vi "03 DPT Channel Tester.vi"() -> ()   [LabVIEW 2009]
uses:
  Hybrid Water Heater/Experiments/Sensor.ctl
  Global Test Variables DPT.vi
  <vilib>/Analysis/NI_AALBase.lvlib
panel:
  out "Output Data (Numbers Only)":dbl[](array[numeric]) format="%.2e"
  in  "Panel 4":T1[][](array[typedef])=[[{"Mean"=0.0, " St Dev."=0.0, "Color Box"=8585007}, {"Mean"=0.0, " St Dev."=0.0, "Color Box"=8585007}, {"Mean"=0.0, " St Dev."=0.0, "Color Box"=8585007}, {"Mean"=0.0, " St Dev."=0.0, "Color Box"=8585007}, {"Mean"=0.0, " St Dev."=0.0, "Color Box"=8585007}, {"Mean"=0.0, " St Dev."=0.0, "Color Box"=8585007}], [{"Mean"=0.0, " St Dev."=0.0, "Color Box"=8585007}, {"Mean"=0.0, " St Dev."=0.0, "Color Box"=8585007}, {"Mean"=0.0, " St Dev."=0.0, "Color Box"=8585007}, {"Mean"=0.0, " St Dev."=0.0, "Color Box"=8585007}, {"Mean"=0.0, " St Dev."=0.0, "Color Box"=8585007}, {"Mean"=0.0, " St Dev."=0.0, "Color Box"=8585007}], [{"Mean"=0.0, " St Dev."=0.0, "Color Box"=8585007}, {"Mean"=0.0, " St Dev."=0.0, "Color Box"=8585007}, {"Mean"=0.0, " St Dev."=0.0, "Color Box"=8585007}, {"Mean"=0.0, " St Dev."=0.0, "Color Box"=8585007}, {"Mean"=0.0, " St Dev."=0.0, "Color Box"=8585007}, {"Mean"=0.0, " St Dev."=0.0, "Color Box"=8585007}]]
  in  "Agilent Reference":refnum<visa-resource-name>="AGILENT-34980A"
  in  "Analog Min OK":dbl=100.0
  in  "Analog Max OK":dbl=400.0
  in  "StDev Thresh":dbl=0.2
  in  "TC Min OK Val":dbl=20.0
  in  "TC Max OK Val":dbl=400.0
  out "Analog":T1[](array[typedef])=[{"Mean"=0.0, " St Dev."=0.0, "Color Box"=8585007}, {"Mean"=0.0, " St Dev."=0.0, "Color Box"=8585007}, {"Mean"=0.0, " St Dev."=0.0, "Color Box"=8585007}]
  in  "Panel 3":T1[][](array[typedef])=[[{"Mean"=0.0, " St Dev."=0.0, "Color Box"=8585007}, {"Mean"=0.0, " St Dev."=0.0, "Color Box"=8585007}, {"Mean"=0.0, " St Dev."=0.0, "Color Box"=8585007}, {"Mean"=0.0, " St Dev."=0.0, "Color Box"=8585007}, {"Mean"=0.0, " St Dev."=0.0, "Color Box"=8585007}, {"Mean"=0.0, " St Dev."=0.0, "Color Box"=8585007}], [{"Mean"=0.0, " St Dev."=0.0, "Color Box"=8585007}, {"Mean"=0.0, " St Dev."=0.0, "Color Box"=8585007}, {"Mean"=0.0, " St Dev."=0.0, "Color Box"=8585007}, {"Mean"=0.0, " St Dev."=0.0, "Color Box"=8585007}, {"Mean"=0.0, " St Dev."=0.0, "Color Box"=8585007}, {"Mean"=0.0, " St Dev."=0.0, "Color Box"=8585007}], [{"Mean"=0.0, " St Dev."=0.0, "Color Box"=8585007}, {"Mean"=0.0, " St Dev."=0.0, "Color Box"=8585007}, {"Mean"=0.0, " St Dev."=0.0, "Color Box"=8585007}, {"Mean"=0.0, " St Dev."=0.0, "Color Box"=8585007}, {"Mean"=0.0, " St Dev."=0.0, "Color Box"=8585007}, {"Mean"=0.0, " St Dev."=0.0, "Color Box"=8585007}]]
  in  "Panel 2":T1[][](array[typedef])=[[{"Mean"=0.0, " St Dev."=0.0, "Color Box"=8585007}, {"Mean"=0.0, " St Dev."=0.0, "Color Box"=8585007}, {"Mean"=0.0, " St Dev."=0.0, "Color Box"=8585007}, {"Mean"=0.0, " St Dev."=0.0, "Color Box"=8585007}, {"Mean"=0.0, " St Dev."=0.0, "Color Box"=8585007}, {"Mean"=0.0, " St Dev."=0.0, "Color Box"=8585007}], [{"Mean"=0.0, " St Dev."=0.0, "Color Box"=8585007}, {"Mean"=0.0, " St Dev."=0.0, "Color Box"=8585007}, {"Mean"=0.0, " St Dev."=0.0, "Color Box"=8585007}, {"Mean"=0.0, " St Dev."=0.0, "Color Box"=8585007}, {"Mean"=0.0, " St Dev."=0.0, "Color Box"=8585007}, {"Mean"=0.0, " St Dev."=0.0, "Color Box"=8585007}], [{"Mean"=0.0, " St Dev."=0.0, "Color Box"=8585007}, {"Mean"=0.0, " St Dev."=0.0, "Color Box"=8585007}, {"Mean"=0.0, " St Dev."=0.0, "Color Box"=8585007}, {"Mean"=0.0, " St Dev."=0.0, "Color Box"=8585007}, {"Mean"=0.0, " St Dev."=0.0, "Color Box"=8585007}, {"Mean"=0.0, " St Dev."=0.0, "Color Box"=8585007}]]
  in  "Panel 1":T1[][](array[typedef])=[[{"Mean"=0.0, " St Dev."=0.0, "Color Box"=8585007}, {"Mean"=0.0, " St Dev."=0.0, "Color Box"=8585007}, {"Mean"=0.0, " St Dev."=0.0, "Color Box"=8585007}, {"Mean"=0.0, " St Dev."=0.0, "Color Box"=8585007}, {"Mean"=0.0, " St Dev."=0.0, "Color Box"=8585007}, {"Mean"=0.0, " St Dev."=0.0, "Color Box"=8585007}], [{"Mean"=0.0, " St Dev."=0.0, "Color Box"=8585007}, {"Mean"=0.0, " St Dev."=0.0, "Color Box"=8585007}, {"Mean"=0.0, " St Dev."=0.0, "Color Box"=8585007}, {"Mean"=0.0, " St Dev."=0.0, "Color Box"=8585007}, {"Mean"=0.0, " St Dev."=0.0, "Color Box"=8585007}, {"Mean"=0.0, " St Dev."=0.0, "Color Box"=8585007}], [{"Mean"=0.0, " St Dev."=0.0, "Color Box"=8585007}, {"Mean"=0.0, " St Dev."=0.0, "Color Box"=8585007}, {"Mean"=0.0, " St Dev."=0.0, "Color Box"=8585007}, {"Mean"=0.0, " St Dev."=0.0, "Color Box"=8585007}, {"Mean"=0.0, " St Dev."=0.0, "Color Box"=8585007}, {"Mean"=0.0, " St Dev."=0.0, "Color Box"=8585007}]]
  in  "Num Samples":i32=5
  in  "error in (no error)":errorcluster
  in  "Test DAQ":bool
  in  "OK":bool
  # "DPT Pannel Channel Tester"
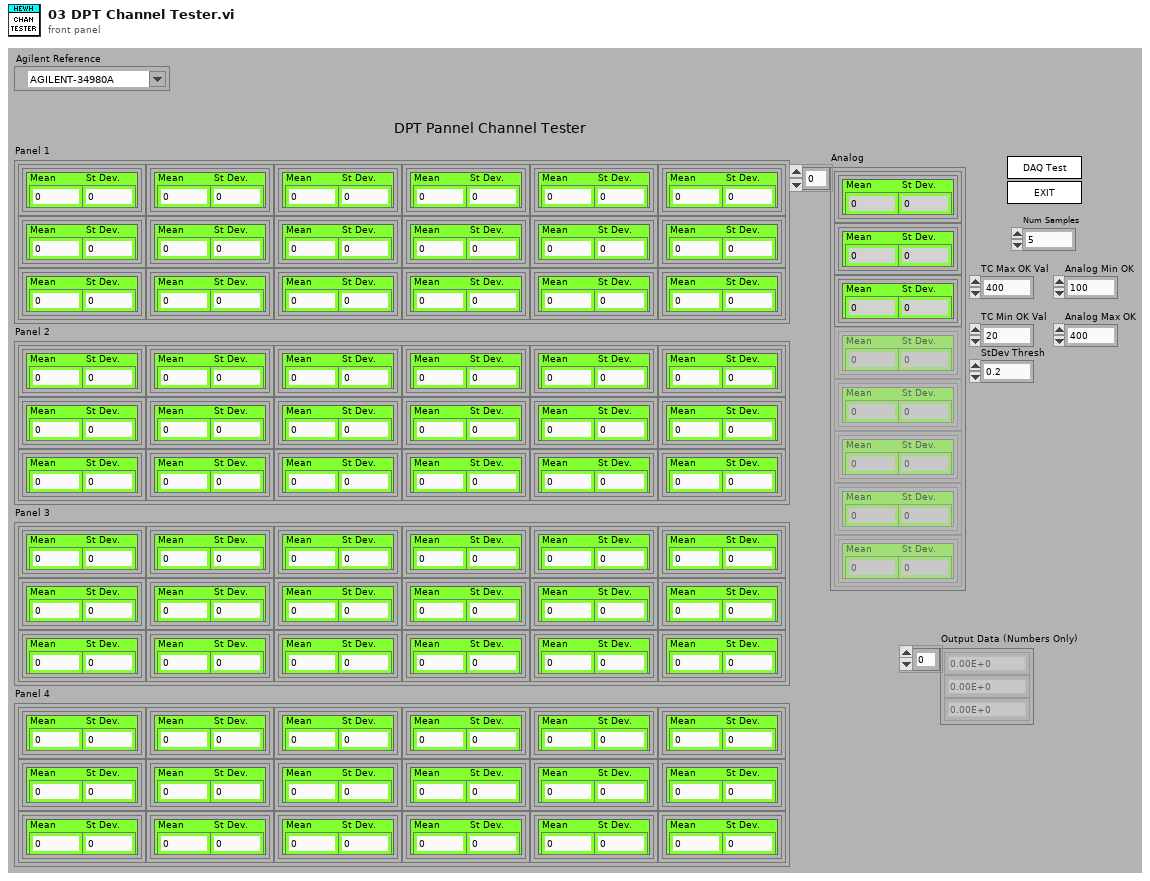
[diagram p1: front panel]
types:
  T1 = typedef "Sensor.ctl" = cluster{"Mean":dbl, " St Dev.":dbl, "Color Box":u32}
  T2 = enum32{"invalid app kind", "Development System", "Run Time System", "Student Edition", "Embedded LabVIEW", "Evaluation", "Custom"}
  T3 = enum32{"Invalid", "Standard", "Closed", "Hidden", "Minimized", "Maximized"}
  T4 = enum16{"100 mV", "1 V", "10 V", "100 V", "300 V", "Auto", "Minimum", "Maximum"}
  T5 = enum16{"B-Type", "E-Type", "J-Type", "K-Type", "N-Type", "R-Type", "S-Type", "T-Type"}
  T6 = cluster{"Core":cluster{"Current VI Reference":refnum<vi>, "Close Panel on Exit?":bool}, "Num Samples":i32, "Agilent Reference":refnum<visa-resource-name>, "Test Data Array":T1[]}
  T7 = cluster{"Current VI Reference":refnum<vi>, "Close Panel on Exit?":bool}
  T8 = typedef "DPT Global Type.ctl" = cluster{"Test Setup":cluster{"3010 resistor":dbl, "Temp Cal":dbl, "Temp Coeff":dbl, "Power On Threshold":dbl, "MA Filter Size":i32, "Weight Offset":dbl, "3011 resistor":dbl, "Gas Enabled":bool, "1020 resistor":dbl, "Scale Com":dbl, "W. Samps":i32}, "Agilent Setup":cluster{"Scale Channel":string, "TC Channels":string, "VDC Discrete Channels":string, "RH Chan":string, "Temp Chan":string, "Tscale Channel":string, "RDB Channel":string, "Gas Temperature":string, "Gas Pressure":string, "Barometric Pressure":string, "Gas Feedback Chan":string}, "Directories":cluster{"Work File Directory":path, "Save File Directory":path, "Library Directory":path, "Data Backup Directory":path}, "Test Information":cluster{"Model:":string, "Temperature:":string, "Engineer:":string, "Technician:":string, "Comments:":string, "Unit:":string, "TR Number:":string, "Test Number:":string, "Test Station:":string, "Empty Dryer Cold Weight:":dbl, "Serial Number:":string, "Build:":string, "Dryer Type":string, "Humidity":string, "Test Title per TR:":string}}
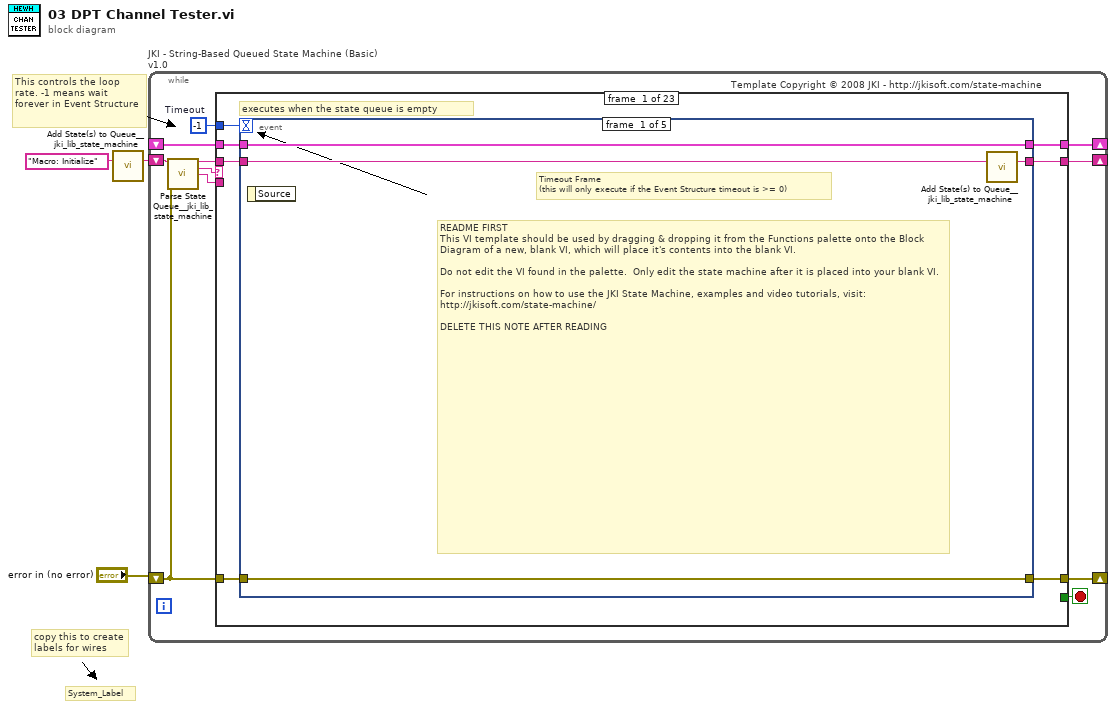
[diagram p0: block diagram]
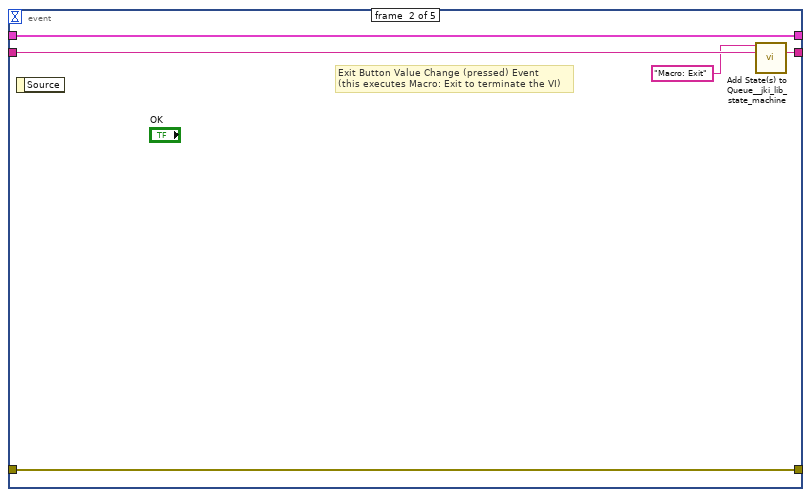
[diagram p2: hidden frame]
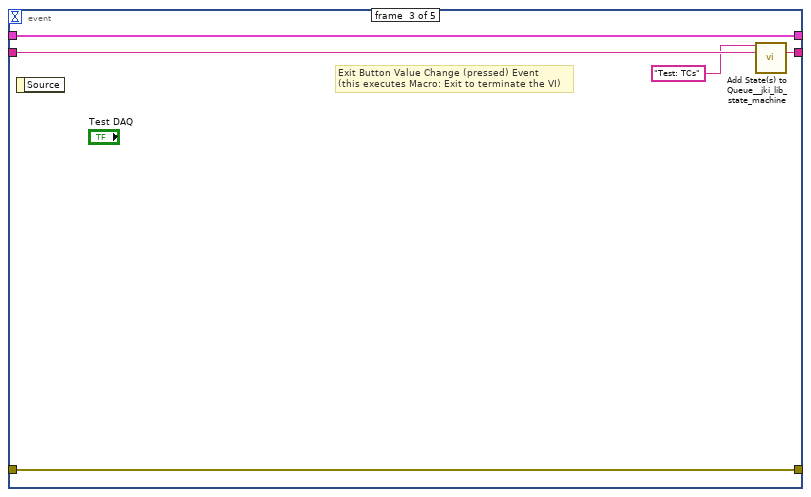
[diagram p3: hidden frame]
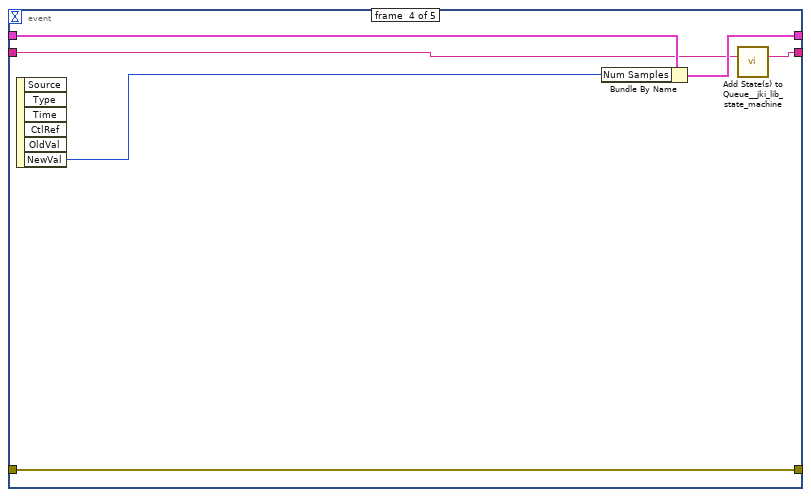
[diagram p4: hidden frame]
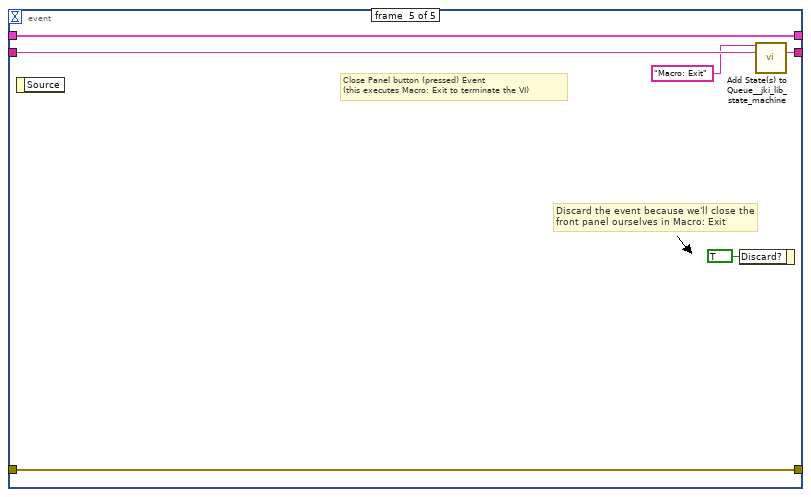
[diagram p5: hidden frame]
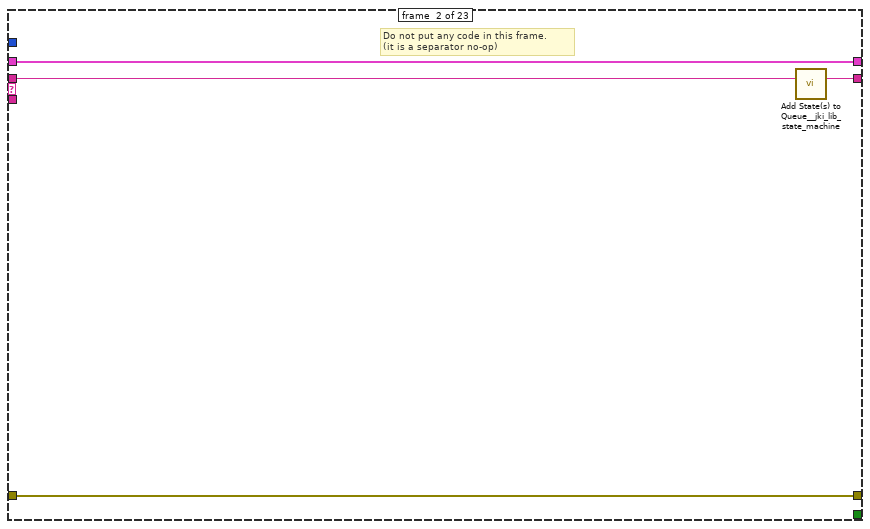
[diagram p6: hidden frame]
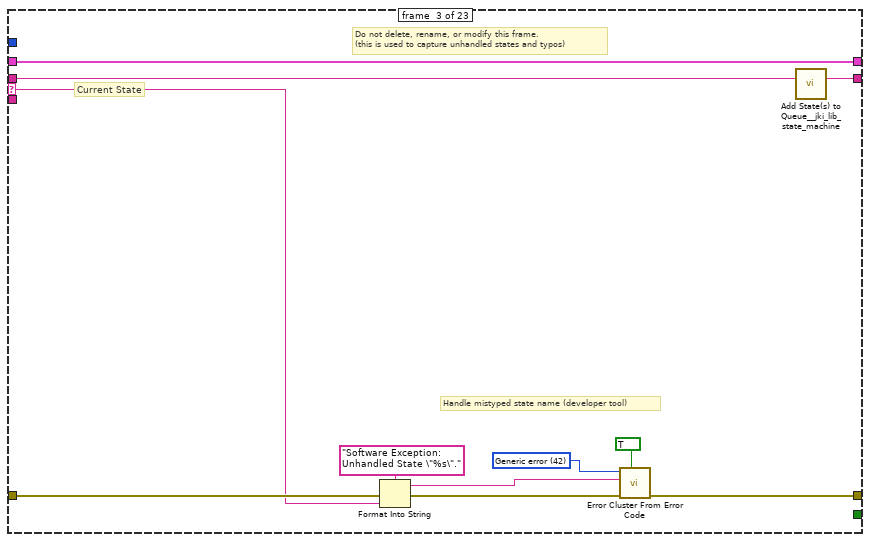
[diagram p7: hidden frame]
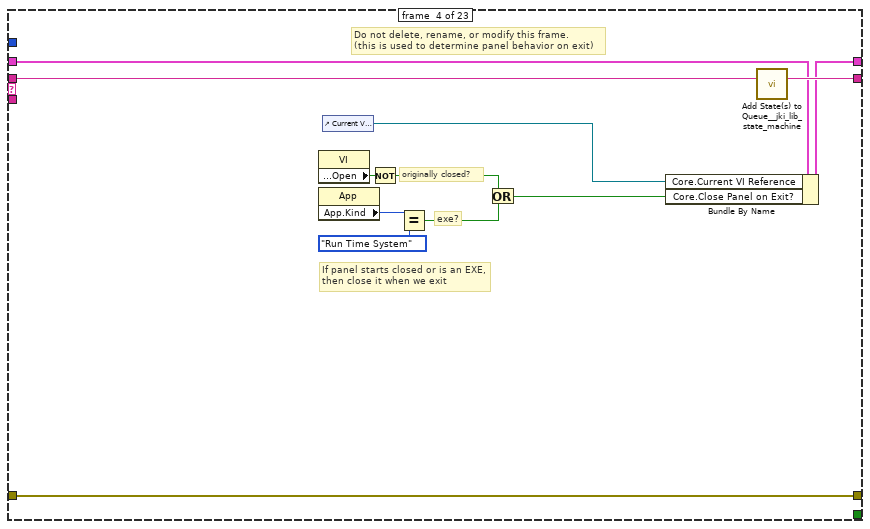
[diagram p8: hidden frame]
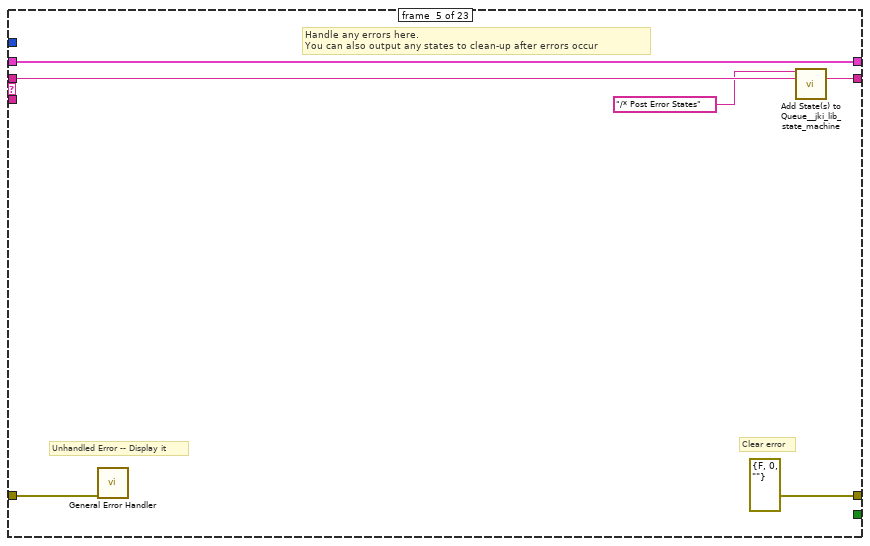
[diagram p9: hidden frame]
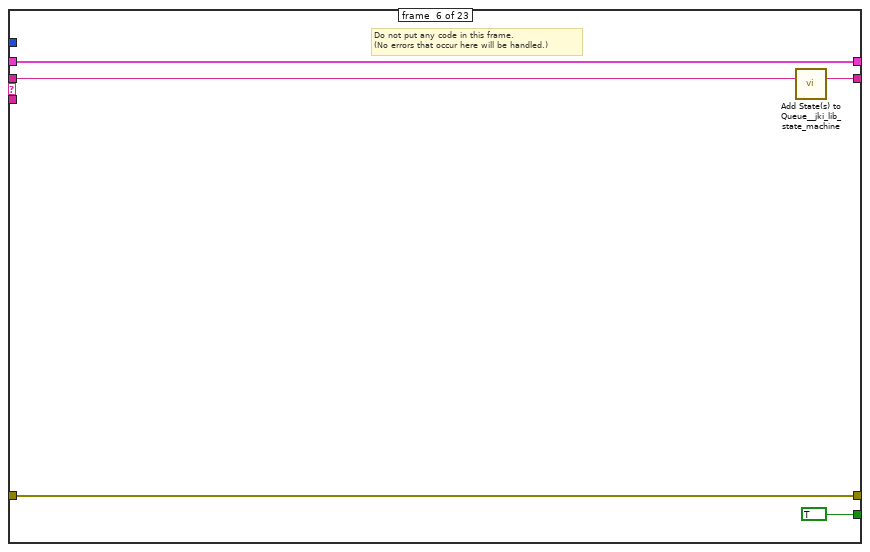
[diagram p10: hidden frame]
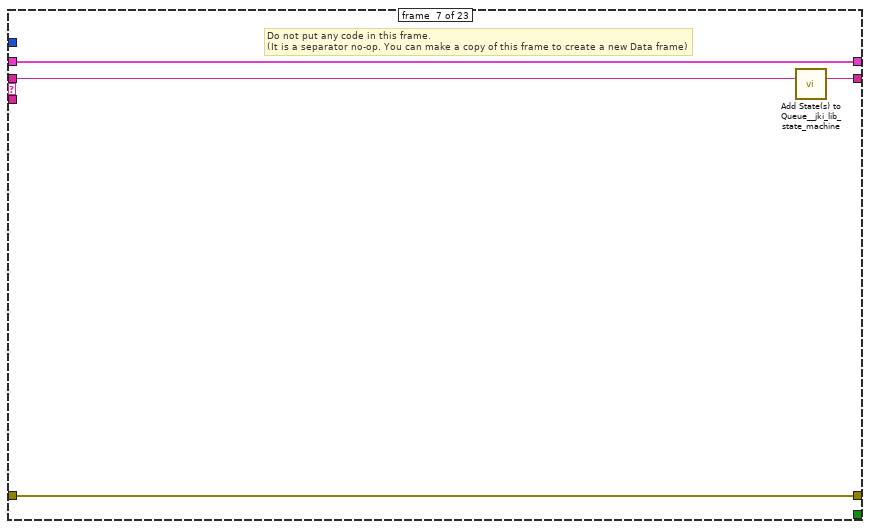
[diagram p11: hidden frame]
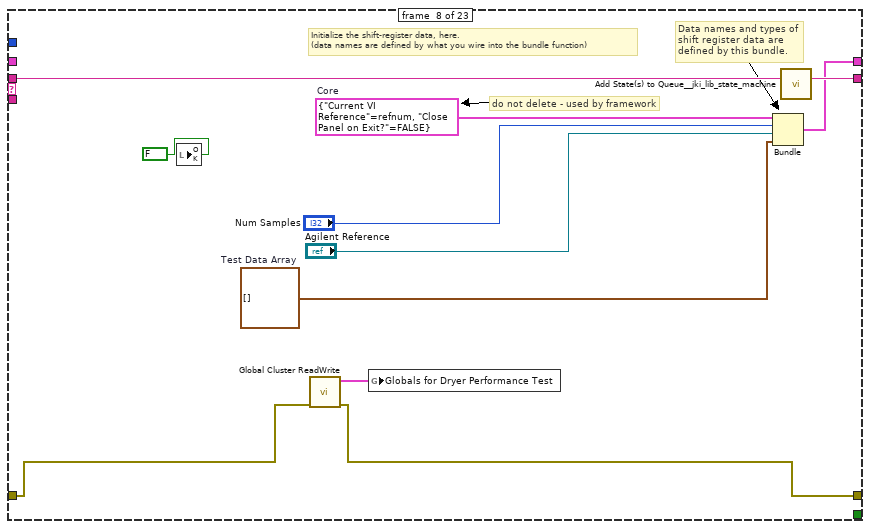
[diagram p12: hidden frame]
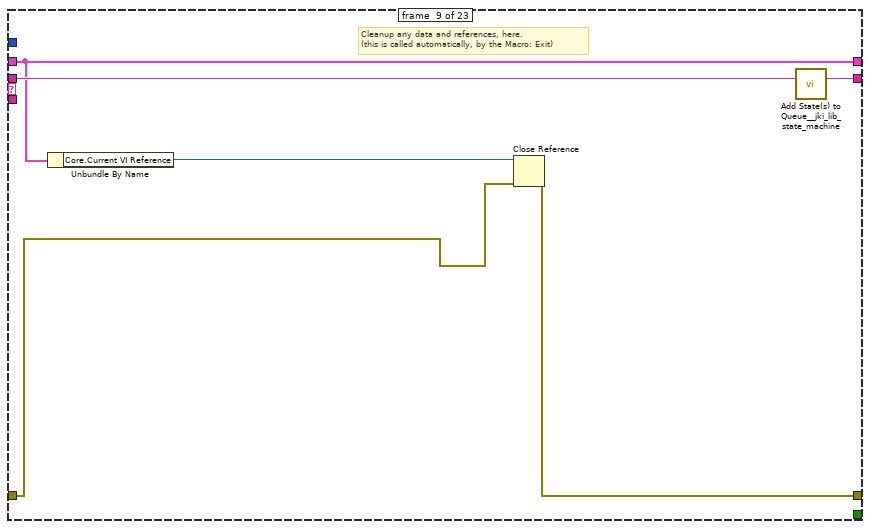
[diagram p13: hidden frame]
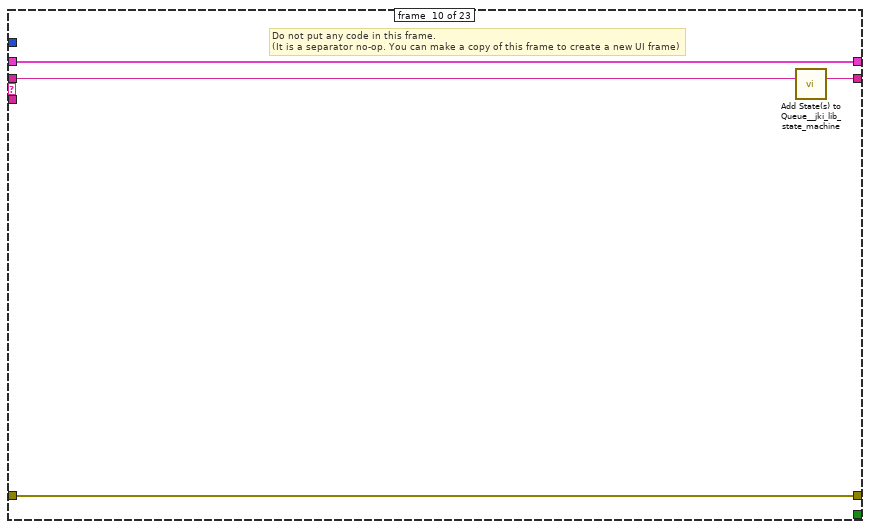
[diagram p14: hidden frame]
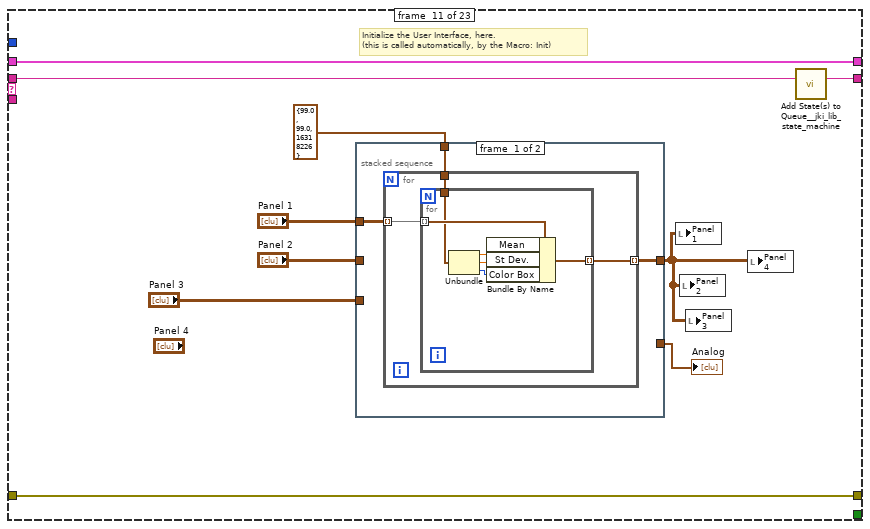
[diagram p15: hidden frame]
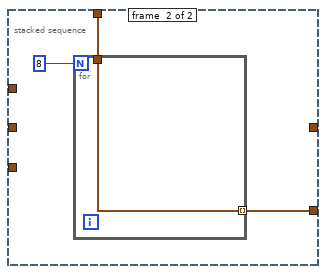
[diagram p16: hidden frame]
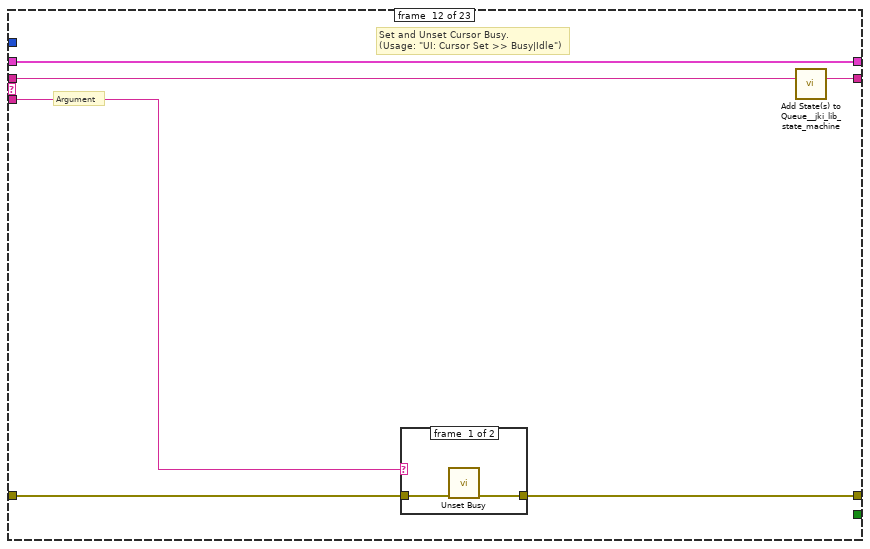
[diagram p17: hidden frame]
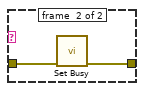
[diagram p18: hidden frame]
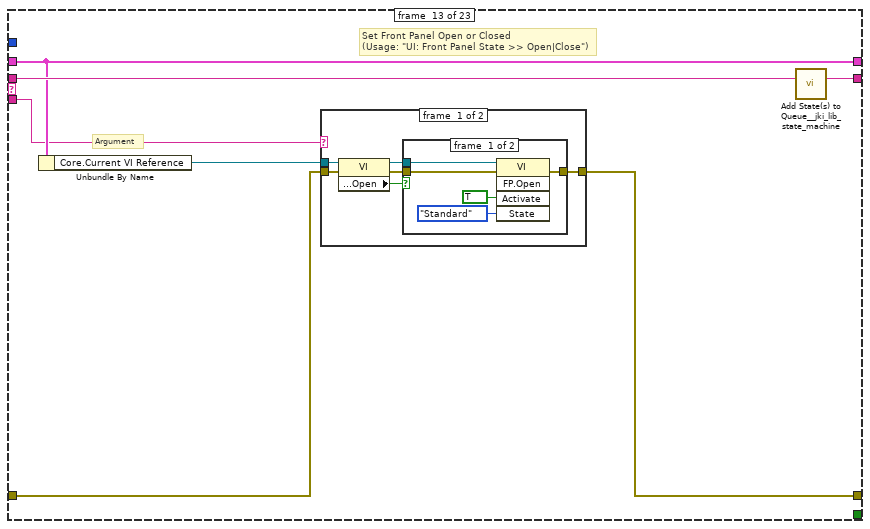
[diagram p19: hidden frame]
diagram:
  # "copy this to create labels for wires"
  # "This controls the loop rate. -1 means wait forever in Event Structure"
  # "System_Label"
  n1 = call <vilib>:"Add State(s) to Queue__jki_lib_state_machine.vi"("State(s) in (\"\")"="Macro: Initialize") -> ("States Out"=w3:string)  [unwired: 14 in]
  n2 = while "JKI - String-Based Queued State Machine (Basic) v1.0" {
    shift-right: [w7] -> _
    shift-left: _ -> [w6]
    shift-right: [w10] -> _
    shift-left: "error in (no error)" -> [w4]
    shift-right: [w9] -> _
    shift-left: w3 -> [w11]
    stop <- w8 stop-if-true
    w5 = -1  # Timeout
    # "Template Copyright © 2008 JKI - http://jkisoft.com/state-machine"
    n3 = call <vilib>:"Parse State Queue__jki_lib_state_machine.vi"("State Queue"=w11, "Error In (no error)"=w4) -> ("Remaining States"=w13:string, "Current State"=w14:string, "Arguments"=w12:string)  [unwired: 11 in]
    n4 = case shown="\"Init: Agilent\"" w14 {
      selector: w14 -> [_ _ w52 _ _ _ _ _ _ _ _ _ _ _ _ _ _ _ _ _ _ _ _]
      tunnel: w13 -> [w21 w51 w56 w74 w80 w85 w89 w100 w106 w110 w120 w142 w153 w179 w184 w210 w220 w224 w229 w233 w244 w264 w343]
      tunnel: w12 -> [_ _ _ _ _ _ _ _ _ _ _ w137 w147 _ _ _ _ _ _ _ _ _ _]
      tunnel: w6 -> [w19 w48 w54 w65 w77 w83 w86 _ w102 w107 w118 w140 w149 w176 w181 w199 w217 w221 w227 w230 w242 w261 w340]
      tunnel: [w18 w49 w58 w71 errorcluster {"status"=FALSE, "code"=0, "source"=""} ("error out") w82 w87 w90 w103 w108 w117 w138 w150 w177 w182 w197 w218 w222 w225 w231 w234 w262 w341] -> w10
      tunnel: w4 -> [w17 w49 w57 w71 w76 w82 w87 w91 w101 w108 w117 w139 w151 w177 w182 w198 w218 w222 w225 w231 w236 w262 w341]
      tunnel: [w20 w50 w55 w73 w79 w84 w88 w99 w105 w109 w119 w141 w152 w178 w183 w209 w219 w223 w228 w232 w243 w263 w342] -> w9
      tunnel: [_ _ _ _ _ TRUE _ _ _ _ _ _ _ _ _ _ _ _ _ _ _ _ _] -> w8
      tunnel: [w16 w48 w54 w72 w77 w83 w86 w98 w102 w107 w118 w140 w149 w176 w181 w199 w217 w221 w227 w230 w240 w261 w340] -> w7
      tunnel: w5 -> [w15 _ _ _ _ _ _ _ _ _ _ _ _ _ _ _ _ _ _ _ _ _ _]
      frame #0 {
        # "executes when the state queue is empty"
        n5 = event shown="[2] \"Test DAQ\": Value Change" {
          selector: _ -> [_ _ _ _ _]
          dyn-events: _ -> [_ _ _ _ _]
          timeout: w15 -> [_ _ _ _ _]
          tunnel: w21 -> [w25 w30 w35 w39 w47]
          tunnel: [w24 w29 w34 w38 w46] -> w20
          tunnel: w19 -> [w22 w27 w32 w41 w44]
          tunnel: [w23 w28 w33 w37 w45] -> w18
          tunnel: w17 -> [w23 w28 w33 w37 w45]
          tunnel: [w22 w27 w32 w40 w44] -> w16
          event #0 {
            # "README FIRST\nThis VI template should be used by dragging & dropping it from the Functions palette onto the Block Diagram of a new, blank VI, which will place it's contents into the blank VI.\n\nDo not edit the VI found in the palette.  Only edit the state machine after it is placed into your blank VI.\n\nFor instructions on how to use the JKI State Machine, examples and video tutorials, visit:\nhttp://jkisoft.com/state-machine/\n\nDELETE THIS NOTE AFTER READING"
            # "Timeout Frame\n(this will only execute if the Event Structure timeout is >= 0)"
            n6 = event-data() -> ()  [unwired: 1 in, 1 out]
            n7 = call <vilib>:"Add State(s) to Queue__jki_lib_state_machine.vi"("State(s) in (\"\")"=w25) -> ("States Out"=w24:string)  [unwired: 14 in]
          }
          event #1 {
            # "Exit Button Value Change (pressed) Event\n(this executes Macro: Exit to terminate the VI)"
            n8 = event-data() -> ()  [unwired: 1 in, 1 out]
            n9 = call <vilib>:"Add State(s) to Queue__jki_lib_state_machine.vi"("State(s) in Front (\"\")"="Macro: Exit", "State(s) in (\"\")"=w30) -> ("States Out"=w29:string)  [unwired: 13 in]
          }
          event #2 {
            # "Exit Button Value Change (pressed) Event\n(this executes Macro: Exit to terminate the VI)"
            n10 = event-data() -> ()  [unwired: 1 in, 1 out]
            n11 = call <vilib>:"Add State(s) to Queue__jki_lib_state_machine.vi"("State(s) in Front (\"\")"="Test: TCs", "State(s) in (\"\")"=w35) -> ("States Out"=w34:string)  [unwired: 13 in]
          }
          event #3 {
            n12 = event-data() -> ("NewVal"=w36:i32)  [unwired: 1 in, 5 out]
            n13 = Bundle By Name(cluster=w41, "Num Samples"=w36) -> (w40:T6)
            n14 = call <vilib>:"Add State(s) to Queue__jki_lib_state_machine.vi"("State(s) in (\"\")"=w39) -> ("States Out"=w38:string)  [unwired: 14 in]
          }
          event #4 {
            # "Discard the event because we'll close the front panel ourselves in Macro: Exit"
            # "Close Panel button (pressed) Event\n(this executes Macro: Exit to terminate the VI)"
            n15 = event-data() -> ()  [unwired: 1 in, 1 out]
            n16 = event-data("Discard?"=TRUE) -> ()  [unwired: 1 in, 1 out]
            n17 = call <vilib>:"Add State(s) to Queue__jki_lib_state_machine.vi"("State(s) in Front (\"\")"="Macro: Exit", "State(s) in (\"\")"=w47) -> ("States Out"=w46:string)  [unwired: 13 in]
          }
        }
      }
      frame #1 {
        # "Do not put any code in this frame.\n(it is a separator no-op)"
        n18 = call <vilib>:"Add State(s) to Queue__jki_lib_state_machine.vi"("State(s) in (\"\")"=w51) -> ("States Out"=w50:string)  [unwired: 14 in]
      }
      frame #2 {
        w61 = 42 items=["No error", "Argument error", "Memory is full", "Out of zone", "End of file", "File already open", "Generic file I/O error", "File not found", "File permission error", "Disk is full", "Duplicate path", "Too many files open", "System feature not enabled", "Resource file not found", "Cannot add resource", "Resource not found", "Image not found", "Image memory error", "Pen does not exist", "Config type invalid", "Config token not found", "Config parse error", "Config memory error", "Bad external code format", "Bad external code offset", "External code not present", "Null window", "Destroy window error", "Null menu", "Print aborted", "Bad print record", "Print driver error", "Windows error during printing", "Memory error during printing", "Print dialog error", "Generic print error", "Invalid device refnum", "Device not found", "Device parameter error", "Device unit error", "Cannot open device", "Device call aborted", "Generic error", "Cancelled by user", "Object ID too low", "Object ID too high", "Object not in heap", "Unknown heap", "Unknown object (invalid DefProc)", "Unknown object (DefProc not in table)", "Message out of range", "Invalid (null) method", "Unknown message", "Manager call not supported", "Bad address", "Network operation in progress", "Network operation timed out", "Connection is busy", "Network attribute not supported", "Network error", "Address in use", "System out of memory", "Connection aborted", "Connection refused", "Not connected", "Already connected", "Connection closed", "Initialization error (interapplication manager)", "Bad occurrence", "Wait on unbound occurrence handler", "Occurrence queue overflow", "Datalog type conflict", "Unused", "Unrecognized type (interapplication manager)", "Memory corrupt", "Failed to make temporary DLL", "Old CIN version", "Drag socket not found", "Failed to load drop-object", "Failed to register OLE object", "Failed to release OLE object", "Format specifier type mismatch", "Unknown format specifier", "Too few format specifiers", "Too many format specifiers", "Scan failed", "Newer CIN version", "Error converting to variant", "Runtime menu error", "Password tampered", "Variant attribute not found", "Incompatible variant data type", "Event data is not available", "Event Store is not present", "Occurrence is not found", "Event Queue is not created", "Event info is not available", "Refnum passed is NULL", "Error retrieving Class GUID", "Error retrieving CoClass GUID", "Error retrieving TypeLib GUID.", "Bad built application magic bytes.", "Specific driver is different from the specific driver associated with the Logical Name.", "There is no session opened to the class driver.", "Max Error", "MAX - Error with config objects", "MAX - Error loading configuration", "MAX - Group not supported"]
        # "Current State"
        # "Do not delete, rename, or modify this frame.\n(this is used to capture unhandled states and typos)"
        # "Handle mistyped state name (developer tool)"
        n19 = Format Into String(format string="Software Exception: Unhandled State \"%s\"." ("message"), error in=w57, w52) -> (resulting string=w60:string, error out=w59:errorcluster)  [unwired: 1 in]
        n20 = call <vilib>:"Error Cluster From Error Code.vi"("show call chain? (False)"=TRUE, "error in (no error)"=w59, "error message (\"\")"=w60, "error code (0)"=w61) -> ("error out"=w58:errorcluster)  [unwired: 5 in]
        n21 = call <vilib>:"Add State(s) to Queue__jki_lib_state_machine.vi"("State(s) in (\"\")"=w56) -> ("States Out"=w55:string)  [unwired: 14 in]
      }
      frame #3 {
        # "Do not delete, rename, or modify this frame.\n(this is used to determine panel behavior on exit)"
        # "originally closed?"
        # "exe?"
        # "If panel starts closed or is an EXE, then close it when we exit"
        n22 = property class="VI"() -> ("Front Panel.Open"=w70:bool)  [unwired: 2 in, 2 out]
        n23 = property class="App"() -> ("App.Kind"=w69:T2)  [unwired: 2 in, 2 out]
        n24 = control-ref of="Current VI Reference"() -> (w63:refnum<vi>)
        n25 = Not(x=w70) -> (.not. x?=w67:bool)
        n26 = Equal?(x=w69, y=T2."Run Time System" ("Application:Kind")) -> (x = y?=w66:bool)
        n27 = Or(x=w67, y=w66) -> (x .or. y?=w64:bool)
        n28 = Bundle By Name(cluster=w65, "Core.Current VI Reference"=w63, "Core.Close Panel on Exit?"=w64) -> (w72:T6)
        n29 = call <vilib>:"Add State(s) to Queue__jki_lib_state_machine.vi"("State(s) in (\"\")"=w74) -> ("States Out"=w73:string)  [unwired: 14 in]
      }
      frame #4 {
        # "Unhandled Error -- Display it"
        # "Handle any errors here.\nYou can also output any states to clean-up after errors occur"
        # "Clear error"
        n30 = call <vilib>:"General Error Handler.vi"("error in (no error)"=w76) -> ()  [unwired: 10 in, 5 out]
        n31 = call <vilib>:"Add State(s) to Queue__jki_lib_state_machine.vi"("State(s) in Front (\"\")"="/* Post Error States", "State(s) in (\"\")"=w80) -> ("States Out"=w79:string)  [unwired: 13 in]
      }
      frame #5 {
        # "Do not put any code in this frame.\n(No errors that occur here will be handled.)"
        n32 = call <vilib>:"Add State(s) to Queue__jki_lib_state_machine.vi"("State(s) in (\"\")"=w85) -> ("States Out"=w84:string)  [unwired: 14 in]
      }
      frame #6 {
        # "Do not put any code in this frame.\n(It is a separator no-op. You can make a copy of this frame to create a new Data frame)"
        n33 = call <vilib>:"Add State(s) to Queue__jki_lib_state_machine.vi"("State(s) in (\"\")"=w89) -> ("States Out"=w88:string)  [unwired: 14 in]
      }
      frame #7 {
        w94 = T1[] []  # Test Data Array
        w97 = T7 {"Current VI Reference"=refnum, "Close Panel on Exit?"=FALSE}  # Core
        # "do not delete - used by framework"
        # "Data names and types of shift register data are defined by this bundle."
        # "Initialize the shift-register data, here.\n(data names are defined by what you wire into the bundle function)"
        n34 = local write "OK"(FALSE ("OK")) -> ()
        n35 = call "Global Cluster ReadWrite.vi"("error in (no error)"=w91) -> ("error out"=w90:errorcluster, "Test Config Out"=w92:T8)  [unwired: 9 in]
        n36 = global write "Global Test Variables DPT.vi" "Globals for Dryer Performance Test"(w92) -> ()
        n37 = Bundle("Core"=w97, "Num Samples"="Num Samples", "Agilent Reference"="Agilent Reference", "Test Data Array"=w94) -> (w98:T6)  [unwired: 1 in]
        n38 = call <vilib>:"Add State(s) to Queue__jki_lib_state_machine.vi"("State(s) in (\"\")"=w100) -> ("States Out"=w99:string)  [unwired: 14 in]
      }
      frame #8 {
        # "Cleanup any data and references, here.\n(this is called automatically, by the Macro: Exit)"
        n39 = Unbundle By Name(w102) -> ("Core.Current VI Reference"=w104:refnum<vi>)
        n40 = Close Reference(reference=w104, error in (no error)=w101) -> (error out=w103:errorcluster)
        n41 = call <vilib>:"Add State(s) to Queue__jki_lib_state_machine.vi"("State(s) in (\"\")"=w106) -> ("States Out"=w105:string)  [unwired: 14 in]
      }
      frame #9 {
        # "Do not put any code in this frame.\n(It is a separator no-op. You can make a copy of this frame to create a new UI frame)"
        n42 = call <vilib>:"Add State(s) to Queue__jki_lib_state_machine.vi"("State(s) in (\"\")"=w110) -> ("States Out"=w109:string)  [unwired: 14 in]
      }
      frame #10 {
        # "Initialize the User Interface, here.\n(this is called automatically, by the Macro: Init)"
        n43 = stacked-sequence {
          tunnel: "Panel 1" -> [w123 _]
          tunnel: T1 {"Mean"=99.0, " St Dev."=99.0, "Color Box"=16318226} ("Sensor") -> [w122 w135]
          tunnel: [w121 _] -> w111
          tunnel: "Panel 2" -> [_ _]
          tunnel: "Panel 3" -> [_ _]
          tunnel: [_ w133] -> w112
          frame #0 {
            n44 = for {
              tunnel: w123 -> [w126] mode=indexing
              tunnel: w122 -> [w125]
              tunnel: [w124] -> w121 mode=indexing
              n45 = for {
                tunnel: w126 -> [w132] mode=indexing
                tunnel: w125 -> [w131]
                tunnel: [w127] -> w124 mode=indexing
                n46 = Unbundle(w131) -> ("Mean"=w130:dbl, "St Dev."=w129:dbl, "Color Box"=w128:u32)
                n47 = Bundle By Name(cluster=w132, "Mean"=w130, "St Dev."=w129, "Color Box"=w128) -> (w127:T1)
              }
            }
          }
          frame #1 {
            n48 = for {
              N: 8 -> [_]
              tunnel: w135 -> [w136]
              tunnel: [w136] -> w133 mode=indexing
            }
          }
        }
        "Analog" <- w112
        n49 = local write "Panel 1"(w111) -> ()
        n50 = local write "Panel 2"(w111) -> ()
        n51 = local write "Panel 3"(w111) -> ()
        n52 = local write "Panel 4"(w111) -> ()
        n53 = call <vilib>:"Add State(s) to Queue__jki_lib_state_machine.vi"("State(s) in (\"\")"=w120) -> ("States Out"=w119:string)  [unwired: 14 in]
      }
      frame #11 {
        # "Argument"
        # "Set and Unset Cursor Busy.\n(Usage: \"UI: Cursor Set >> Busy|Idle\")"
        n54 = case shown="\"Idle\", Default" w137 {
          tunnel: w139 -> [w144 w146]
          tunnel: [w143 w145] -> w138
          frame #0 {
            n55 = call <vilib>:"Unset Busy.vi"("error in (no error)"=w144) -> ("error out"=w143:errorcluster)  [unwired: 10 in]
          }
          frame #1 {
            n56 = call <vilib>:"Set Busy.vi"("error in (no error)"=w146) -> ("error out"=w145:errorcluster)  [unwired: 9 in, 1 out]
          }
        }
        n57 = call <vilib>:"Add State(s) to Queue__jki_lib_state_machine.vi"("State(s) in (\"\")"=w142) -> ("States Out"=w141:string)  [unwired: 14 in]
      }
      frame #12 {
        # "Argument"
        # "Set Front Panel Open or Closed\n(Usage: \"UI: Front Panel State >> Open|Close\")"
        n58 = Unbundle By Name(w149) -> ("Core.Current VI Reference"=w148:refnum<vi>)
        n59 = case shown="\"Close\"" w147 {
          tunnel: w151 -> [w157 w170]
          tunnel: [w159 w171] -> w150
          tunnel: w148 -> [w158 w168]
          frame #0 {
            n60 = property class="VI"(reference=w158, error in=w157) -> (reference out=w155:refnum<vi>, error out=w156:errorcluster, "Front Panel.Open"=w154:bool)
            n61 = case shown="False" w154 {
              tunnel: [w162 w165] -> w159
              tunnel: w156 -> [w161 w165]
              tunnel: w155 -> [w160 _]
              frame #0 {
                n62 = invoke class="VI" method="FP.Open"(reference=w160, error in=w161, "Activate"=TRUE, "State"=T3."Standard") -> (error out=w162:errorcluster)  [unwired: 1 in, 4 out]
              }
              frame #1 {
              }
            }
          }
          frame #1 {
            n63 = property class="VI"(reference=w168, error in=w170) -> (reference out=w167:refnum<vi>, error out=w169:errorcluster, "Front Panel.Open"=w166:bool)
            n64 = case shown="True" w166 {
              tunnel: [w172 w175] -> w171
              tunnel: w169 -> [w172 w174]
              tunnel: w167 -> [_ w173]
              frame #0 {
              }
              frame #1 {
                n65 = invoke class="VI" method="FP.Close"(reference=w173, error in=w174) -> (error out=w175:errorcluster)  [unwired: 1 in, 2 out]
              }
            }
          }
        }
        n66 = call <vilib>:"Add State(s) to Queue__jki_lib_state_machine.vi"("State(s) in (\"\")"=w153) -> ("States Out"=w152:string)  [unwired: 14 in]
      }
      frame #13 {
        # "Do not put any code in this frame.\n(It is a separator no-op. You can make a copy of this frame to create a new Macro frame)"
        n67 = call <vilib>:"Add State(s) to Queue__jki_lib_state_machine.vi"("State(s) in (\"\")"=w179) -> ("States Out"=w178:string)  [unwired: 14 in]
      }
      frame #14 {
        w180 = "Data: Initialize\nInit: Agilent\nInitialize Core Data\nUI: Initialize\nUI: Front Panel State >> Open"  # Data: Initialize Init: Agilent Initialize Core Data UI: Initialize UI: Front Panel State >> Open
        # "Initialization Macro\n(This is called once, when the VI starts)"
        n68 = call <vilib>:"Add State(s) to Queue__jki_lib_state_machine.vi"("State(s) in Front (\"\")"=w180, "State(s) in (\"\")"=w184) -> ("States Out"=w183:string)  [unwired: 13 in]
      }
      frame #15 {
        # "Initialization Macro\n(This is called once, when the VI starts)"
        n69 = global read "Global Test Variables DPT.vi" "Globals for Dryer Performance Test"() -> (w187:T8)
        n70 = Unbundle By Name(w199) -> ("Agilent Reference"=w191:refnum<visa-resource-name>)
        n71 = property class="Instr"(reference=w191, "General Settings:Timeout Value"=u32 10000) -> (reference out=w190:refnum<visa-resource-name>)  [unwired: 1 in, 1 out]
        n72 = call "AG34980A Initialize.vi"("VISA resource name"=w190, "error in (no error)"=w198) -> ("VISA session"=w200:refnum<visa-resource-name>, "error out"=w201:errorcluster)  [unwired: 12 in]
        n73 = Unbundle By Name(w187) -> ("Agilent Setup.VDC Discrete Channels"=w185:string, "Agilent Setup.TC Channels"=w186:string)
        n74 = call "AG34980A Reset.vi"("VISA resource name"=w200, "error in (no error)"=w201) -> ("VISA resource name out"=w204:refnum<visa-resource-name>, "error out"=w202:errorcluster)  [unwired: 12 in]
        n75 = call "AG34980A Configure Thermocouple.vi"("VISA resource name"=w204, "Channel List(empty)"=w186, "Reading Units (0:Celcius)"=enum16{"Celcius", "Fahrenheit", "Kelvin"}."Fahrenheit", "Thermocouple Type (2:J-Type)"=T5."T-Type", "Reference Junction Type (2:Fixed)"=enum16{"Internal", "External", "Fixed"}."Internal", "error in (no error)"=w202, "Ref Junction Temperature (0:Manual)"=enum16{"Manual", "Minimum", "Maximum"}."Minimum") -> ("VISA resource name out"=w205:refnum<visa-resource-name>, "error out"=w203:errorcluster)  [unwired: 7 in]
        n76 = call "AG34980A Configure DC Voltage.vi"("VISA resource name"=w205, "Channel List(empty)"=w185, "Range (5:Auto)"=T4."Auto", "error in (no error)"=w203) -> ("VISA resource name out"=w195:refnum<visa-resource-name>, "error out"=w194:errorcluster)  [unwired: 10 in]
        n77 = Concatenate Strings(w186, "," ("string"), w185) -> (w193:string)
        n78 = call "AG34980A Configure Scan.vi"("VISA resource name"=w195, "Scan List(empty)"=w193, "error in (no error)"=w194) -> ("error out"=w197:errorcluster)  [unwired: 11 in, 1 out]
        n79 = call <vilib>:"Add State(s) to Queue__jki_lib_state_machine.vi"("State(s) in (\"\")"=w210) -> ("States Out"=w209:string)  [unwired: 14 in]
      }
      frame #16 {
        # "Exit Macro\n(This is called once, when the VI exits)"
        n80 = Unbundle By Name(w217) -> ("Core.Close Panel on Exit?"=w216:bool)
        n81 = Select(t="UI: Front Panel State >> Close", s=w216, f="") -> (s? t:f=w213:string)
        n82 = call <vilib>:"Add State(s) to Queue__jki_lib_state_machine.vi"("State(s) in (\"\")"=w213, "State(s) at Back (\"\")"="Data: Cleanup\nExit") -> ("States Out"=w211:string)  [unwired: 13 in]
        n83 = call <vilib>:"Add State(s) to Queue__jki_lib_state_machine.vi"("State(s) in Front (\"\")"=w211, "State(s) in (\"\")"=w220) -> ("States Out"=w219:string)  [unwired: 13 in]
      }
      frame #17 {
        # "Template Separator\n(You can make a copy of, or modify, this frame)"
        n84 = call <vilib>:"Add State(s) to Queue__jki_lib_state_machine.vi"("State(s) in (\"\")"=w224) -> ("States Out"=w223:string)  [unwired: 14 in]
      }
      frame #18 {
        # "Your code here.\n(You can make a copy of, or modify, this frame)"
        n85 = call <vilib>:"Add State(s) to Queue__jki_lib_state_machine.vi"("State(s) in (\"\")"=w229, "State(s) at Back (\"\")"="TestDAQ: Gather\nTestDAQ: Sort\nTestDAQ: Verify" ("State(s) at Back (\"\")")) -> ("States Out"=w228:string)  [unwired: 13 in]
      }
      frame #19 {
        # "Template Separator\n(You can make a copy of, or modify, this frame)"
        n86 = call <vilib>:"Add State(s) to Queue__jki_lib_state_machine.vi"("State(s) in (\"\")"=w233) -> ("States Out"=w232:string)  [unwired: 14 in]
      }
      frame #20 {
        # "Template Separator\n(You can make a copy of, or modify, this frame)"
        n87 = Unbundle By Name(w242) -> ("Agilent Reference"=w238:refnum<visa-resource-name>, "Num Samples"=w237:i32)
        n88 = for {
          N: w237 -> [_]
          tunnel: w238 -> [w249]
          shift-right: [w247] -> w234
          shift-left: w236 -> [w248]
          tunnel: [w246] -> w235 mode=indexing
          n89 = call "AG34980A Initiate.vi"("VISA resource name"=w249, "error in (no error)"=w248) -> ("VISA resource name out"=w252:refnum<visa-resource-name>, "error out"=w254:errorcluster)  [unwired: 12 in]
          n90 = call "AG34980A Fetch.vi"("VISA resource name"=w252, "Numbers Only (T:On)"=TRUE, "error in (no error)"=w254, "Byte Count (1024 bytes)"=2048) -> ("VISA resource name out"=w251:refnum<visa-resource-name>, "Output Data (Numbers Only)"=w246:dbl[], "error out"=w253:errorcluster)  [unwired: 7 in, 2 out]
          "Output Data (Numbers Only)" <- w246
          n91 = call "AG34980A Error Query (Multiple).vi"("VISA resource name"=w251, "error in (no error)"=w253) -> ("error out"=w247:errorcluster)  [unwired: 10 in, 3 out]
        }
        n92 = Transpose 2D Array(2D array=w235) -> (transposed array=w239:dbl[][])
        n93 = for {
          tunnel: w239 -> [w259] mode=indexing
          tunnel: [w256] -> w241 mode=indexing
          n94 = call <vilib>:"Std Deviation and Variance.vi"("X"=w259) -> ("mean"=w258:dbl, "standard deviation"=w257:dbl)  [unwired: 1 in, 1 out]
          n95 = Bundle By Name(cluster=T1 {"Mean"=0.0, " St Dev."=0.0, "Color Box"=5373696} ("Sensor"), "Mean"=w258, "St Dev."=w257) -> (w256:T1)
        }
        n96 = Bundle By Name(cluster=w242, "Test Data Array"=w241) -> (w240:T6)
        n97 = call <vilib>:"Add State(s) to Queue__jki_lib_state_machine.vi"("State(s) in (\"\")"=w244) -> ("States Out"=w243:string)  [unwired: 14 in]
      }
      frame #21 {
        # "Template Separator\n(You can make a copy of, or modify, this frame)"
        n98 = Unbundle By Name(w261) -> ("Test Data Array"=w260:T1[])
        n99 = stacked-sequence {
          tunnel: w260 -> [w270 w288 w306 w322 w332]
          frame #0 {
            n100 = local read "Panel 1"() -> (w267:T1[][])
            n101 = Array Subset(array=w270, index=0, length=6) -> (w269:T1[])
            n102 = Array Subset(array=w270, index=6, length=6) -> (w266:T1[])
            n103 = Array Subset(array=w270, index=12, length=6) -> (w265:T1[])
            n104 = Replace Array Subset(array=w267, new element=w269, index (row)=0) -> (w279:T1[][])  [unwired: 1 in]
            n105 = Replace Array Subset(array=w279, new element=w266, index (row)=1) -> (w277:T1[][])  [unwired: 1 in]
            n106 = Replace Array Subset(array=w277, new element=w265, index (row)=2) -> (w268:T1[][])  [unwired: 1 in]
            n107 = local write "Panel 1"(w268) -> ()
          }
          frame #1 {
            n108 = local read "Panel 2"() -> (w282:T1[][])
            n109 = Array Subset(array=w288, index=20, length=6) -> (w291:T1[])
            n110 = Array Subset(array=w288, index=26, length=6) -> (w287:T1[])
            n111 = Replace Array Subset(array=w282, new element=w291, index (row)=0) -> (w296:T1[][])  [unwired: 1 in]
            n112 = Array Subset(array=w288, index=32, length=6) -> (w286:T1[])
            n113 = Replace Array Subset(array=w296, new element=w287, index (row)=1) -> (w294:T1[][])  [unwired: 1 in]
            n114 = Replace Array Subset(array=w294, new element=w286, index (row)=2) -> (w285:T1[][])  [unwired: 1 in]
            n115 = local write "Panel 2"(w285) -> ()
          }
          frame #2 {
            (unwired) 6 ("length")
            n116 = local read "Panel 3"() -> (w300:T1[][])
            n117 = Array Subset(array=w306, index=40, length=6) -> (w304:T1[])
            n118 = Array Subset(array=w306, index=46) -> (w303:T1[])  [unwired: 1 in]
            n119 = Array Subset(array=w306, index=52, length=6) -> (w299:T1[])
            n120 = Replace Array Subset(array=w300, new element=w304, index (row)=0) -> (w301:T1[][])  [unwired: 1 in]
            n121 = Replace Array Subset(array=w301, new element=w303, index (row)=1) -> (w311:T1[][])  [unwired: 1 in]
            n122 = Replace Array Subset(array=w311, new element=w299, index (row)=2) -> (w302:T1[][])  [unwired: 1 in]
            n123 = local write "Panel 3"(w302) -> ()
          }
          frame #3 {
            (unwired) 6 ("length")
            n124 = local read "Panel 4"() -> (w316:T1[][])
            n125 = Array Subset(array=w322, index=60, length=6) -> (w320:T1[])
            n126 = Array Subset(array=w322, index=66) -> (w319:T1[])  [unwired: 1 in]
            n127 = Array Subset(array=w322, index=72, length=6) -> (w315:T1[])
            n128 = Replace Array Subset(array=w316, new element=w320, index (row)=0) -> (w317:T1[][])  [unwired: 1 in]
            n129 = Replace Array Subset(array=w317, new element=w319, index (row)=1) -> (w327:T1[][])  [unwired: 1 in]
            n130 = Replace Array Subset(array=w327, new element=w315, index (row)=2) -> (w318:T1[][])  [unwired: 1 in]
            n131 = local write "Panel 4"(w318) -> ()
          }
          frame #4 {
            # "Pressures"
            n132 = Array Subset(array=w332, index=80, length=8) -> (w331:T1[])
            n133 = local write "Analog"(w331) -> ()
          }
        }
        n134 = call <vilib>:"Add State(s) to Queue__jki_lib_state_machine.vi"("State(s) in (\"\")"=w264) -> ("States Out"=w263:string)  [unwired: 14 in]
      }
      frame #22 {
        # "Template Separator\n(You can make a copy of, or modify, this frame)"
        n135 = local read "Panel 3"() -> (w337:T1[][])
        n136 = local read "Panel 1"() -> (w339:T1[][])
        n137 = local read "Panel 4"() -> (w335:T1[][])
        n138 = local read "Analog"() -> (w336:T1[])
        n139 = local read "Panel 2"() -> (w338:T1[][])
        n140 = stacked-sequence {
          tunnel: w338 -> [_ w362 _ _ _]
          tunnel: w339 -> [w344 _ _ _ _]
          tunnel: w337 -> [_ _ w378 _ _]
          tunnel: w336 -> [_ _ _ _ w413]
          tunnel: w335 -> [_ _ _ w395 _]
          frame #0 {
            n141 = for {
              tunnel: [w347] -> w345 mode=indexing
              tunnel: w344 -> [w346] mode=indexing
              n142 = for {
                tunnel: [w355] -> w347 mode=indexing
                tunnel: w346 -> [w352] mode=indexing
                n143 = Unbundle By Name(w352) -> ("Mean"=w349:dbl, "St Dev."=w356:dbl)
                n144 = In Range and Coerce(upper limit="TC Max OK Val", x=w349, lower limit="TC Min OK Val") -> (In Range?=w348:bool)  [unwired: 1 out]
                n145 = Less?(x=w356, y="StDev Thresh") -> (x < y?=w354:bool)
                n146 = And(x=w354, y=w348) -> (x .and. y?=w353:bool)
                n147 = Select(t=u32 5373696 ("Color Box"), s=w353, f=u32 16711680 ("Color Box")) -> (s? t:f=w357:u32)
                n148 = Bundle By Name(cluster=w352, "Mean"=w349, "St Dev."=w356, "Color Box"=w357) -> (w355:T1)
              }
            }
            n149 = local write "Panel 1"(w345) -> ()
          }
          frame #1 {
            n150 = for {
              tunnel: w362 -> [w364] mode=indexing
              tunnel: [w363] -> w361 mode=indexing
              n151 = for {
                tunnel: w364 -> [w377] mode=indexing
                tunnel: [w372] -> w363 mode=indexing
                n152 = local read "StDev Thresh"() -> (w369:dbl)
                n153 = local read "TC Min OK Val"() -> (w366:dbl)
                n154 = local read "TC Max OK Val"() -> (w365:dbl)
                n155 = Unbundle By Name(w377) -> ("Mean"=w368:dbl, "St Dev."=w373:dbl)
                n156 = Less?(x=w373, y=w369) -> (x < y?=w371:bool)
                n157 = In Range and Coerce(upper limit=w365, x=w368, lower limit=w366) -> (In Range?=w367:bool)  [unwired: 1 out]
                n158 = And(x=w371, y=w367) -> (x .and. y?=w370:bool)
                n159 = Select(t=u32 5373696 ("Color Box"), s=w370, f=u32 16711680 ("Color Box")) -> (s? t:f=w374:u32)
                n160 = Bundle By Name(cluster=w377, "Mean"=w368, "St Dev."=w373, "Color Box"=w374) -> (w372:T1)
              }
            }
            n161 = local write "Panel 2"(w361) -> ()
          }
          frame #2 {
            n162 = for {
              tunnel: w378 -> [w381] mode=indexing
              tunnel: [w380] -> w379 mode=indexing
              n163 = for {
                tunnel: w381 -> [w394] mode=indexing
                tunnel: [w389] -> w380 mode=indexing
                n164 = local read "TC Min OK Val"() -> (w385:dbl)
                n165 = Unbundle By Name(w394) -> ("Mean"=w384:dbl, "St Dev."=w390:dbl)
                n166 = local read "StDev Thresh"() -> (w386:dbl)
                n167 = local read "TC Max OK Val"() -> (w383:dbl)
                n168 = Less?(x=w390, y=w386) -> (x < y?=w388:bool)
                n169 = In Range and Coerce(upper limit=w383, x=w384, lower limit=w385) -> (In Range?=w382:bool)  [unwired: 1 out]
                n170 = And(x=w388, y=w382) -> (x .and. y?=w387:bool)
                n171 = Select(t=u32 5373696 ("Color Box"), s=w387, f=u32 16711680 ("Color Box")) -> (s? t:f=w391:u32)
                n172 = Bundle By Name(cluster=w394, "Mean"=w384, "St Dev."=w390, "Color Box"=w391) -> (w389:T1)
              }
            }
            n173 = local write "Panel 3"(w379) -> ()
          }
          frame #3 {
            n174 = for {
              tunnel: w395 -> [w398] mode=indexing
              tunnel: [w397] -> w396 mode=indexing
              n175 = for {
                tunnel: w398 -> [w411] mode=indexing
                tunnel: [w406] -> w397 mode=indexing
                n176 = local read "TC Min OK Val"() -> (w402:dbl)
                n177 = Unbundle By Name(w411) -> ("Mean"=w401:dbl, "St Dev."=w407:dbl)
                n178 = local read "StDev Thresh"() -> (w403:dbl)
                n179 = local read "TC Max OK Val"() -> (w400:dbl)
                n180 = Less?(x=w407, y=w403) -> (x < y?=w405:bool)
                n181 = In Range and Coerce(upper limit=w400, x=w401, lower limit=w402) -> (In Range?=w399:bool)  [unwired: 1 out]
                n182 = And(x=w405, y=w399) -> (x .and. y?=w404:bool)
                n183 = Select(t=u32 5373696 ("Color Box"), s=w404, f=u32 16711680 ("Color Box")) -> (s? t:f=w408:u32)
                n184 = Bundle By Name(cluster=w411, "Mean"=w401, "St Dev."=w407, "Color Box"=w408) -> (w406:T1)
              }
            }
            n185 = local write "Panel 4"(w396) -> ()
          }
          frame #4 {
            n186 = for {
              tunnel: w413 -> [w426] mode=indexing
              tunnel: [w421] -> w412 mode=indexing
              n187 = Unbundle By Name(w426) -> ("Mean"=w415:dbl, "St Dev."=w422:dbl)
              n188 = local read "StDev Thresh"() -> (w418:dbl)
              n189 = In Range and Coerce(upper limit="Analog Max OK", x=w415, lower limit="Analog Min OK") -> (In Range?=w414:bool)  [unwired: 1 out]
              n190 = Less?(x=w422, y=w418) -> (x < y?=w420:bool)
              n191 = And(x=w420, y=w414) -> (x .and. y?=w419:bool)
              n192 = Select(t=u32 5373696 ("Color Box"), s=w419, f=u32 16711680 ("Color Box")) -> (s? t:f=w423:u32)
              n193 = Bundle By Name(cluster=w426, "Mean"=w415, "St Dev."=w422, "Color Box"=w423) -> (w421:T1)
            }
            n194 = local write "Analog"(w412) -> ()
          }
        }
        n195 = call <vilib>:"Add State(s) to Queue__jki_lib_state_machine.vi"("State(s) in (\"\")"=w343) -> ("States Out"=w342:string)  [unwired: 14 in]
      }
    }
  }
